vi "StartUp Sequence Open Loop Rev 1.6.vi"() -> ()   [LabVIEW 2017]
uses:
  <vilib>/addons/control/pid/NI_PID_pid.lvlib
  <vilib>/addons/control/pid/pid.llb/PID (DBL).vi
panel:
  in  "Stop":bool
  out "Process variable and Setpoint":cluster{"initial PV":dbl, "SP:":dbl}(graph)
  in  "PID gains":T1={"proportional gain (Kc)"=20.0, "integral time (Ti, min)"=0.008, "derivative time (Td, min)"=0.001} {"derivative time (Td, min)" format="%.3f"; "integral time (Ti, min)" format="%.3f"; "proportional gain (Kc)" format="%.3f"}
  out "Measured RPM:":dbl(slide)=60.754431603254424 scale=0.0..100.0
  in  "Requested RPM:":dbl(slide)=43.790849673202615 min=0.0 max=0.0 scale=0.0..100.0
  out "MV:":dbl(slide)=18.78965245852964 scale=-100.0..100.0
  out "Manipulated variable":i32(graph)
  out "Requested RPM":i32
  out "Waveform Chart":cluster{i32, i32}(graph)
  in  "Set RPM":string
  out "Pump Value 2":string
  in  "Soft Shut Off":bool
  out "Pump Value 1":string
  in  "Send RPM":bool
  in  "Send Command":bool
  in  "Custom Command":string
  out "Startup Success":bool
  in  "Output File":path
  in  "Shut Off":bool
  out "ECU COM Port Out":refnum<visa-resource-name>
  out "Throttle Position":string
  out "Turbine RPM":string
  out "Turbine Temp":string
  out "Error Out":errorcluster
  in  "Error In":errorcluster
  in  "ECU COM Port":refnum<visa-resource-name>
  out "Turbine State":string
  in  "Strt Sqnc":bool
  # "Note: save to a .csv file"
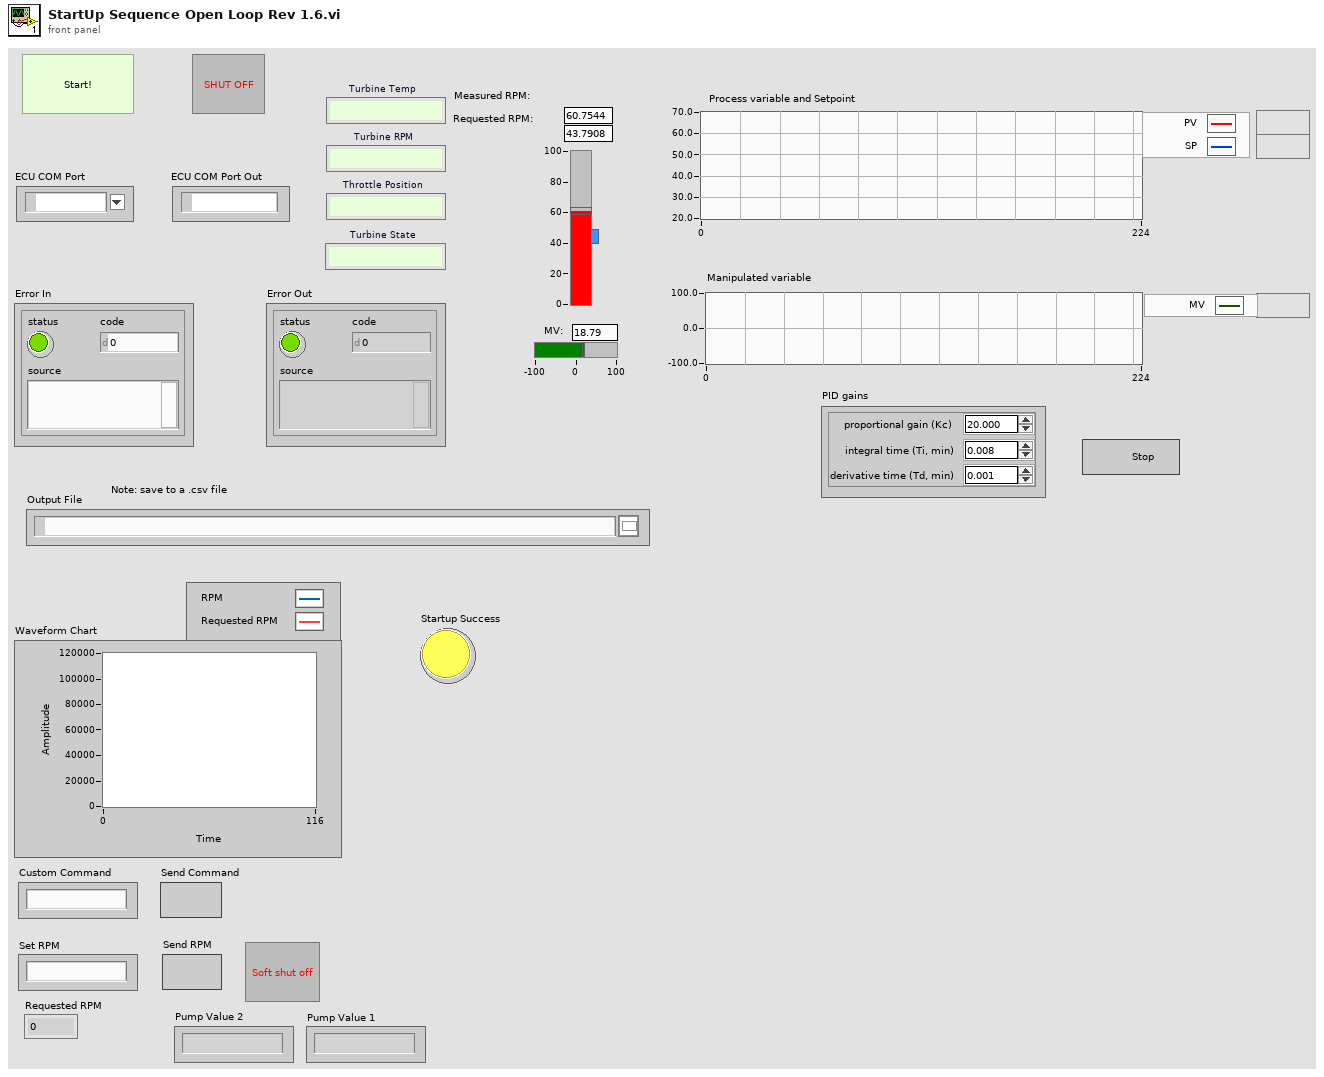
[diagram p1: front panel]
types:
  T1 = cluster{"proportional gain (Kc)":dbl, "integral time (Ti, min)":dbl, "derivative time (Td, min)":dbl}
  T2 = cluster{"Plant Output":dbl, "Requested RPM:":dbl}
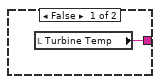
[diagram p4: hidden frame]
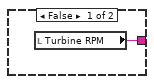
[diagram p5: hidden frame]
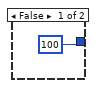
[diagram p7: hidden frame]
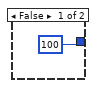
[diagram p8: hidden frame]
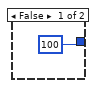
[diagram p9: hidden frame]
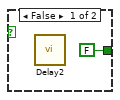
[diagram p11: hidden frame]
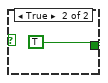
[diagram p12: hidden frame]
diagram:
  w21 = 21 ("Pulse Width")
  w22 = 160 ("Voltage")
  w27 = 16 ("Pulse Width")
  w28 = 160 ("Voltage")
  w18 = 255 ("y")
  w19 = 80 ("y")
  # "NOTE:\nThere are data entry limits\non this input. These may need\nto be deleted in the future"
  # "Disengage Starter Motor"
  # "Starter Motor 55%"
  # "Start button is inside a while loop that doesn't progess until True"
  # "Fuel Pump Mode 2"
  # "GlowPlugOff"
  # "Start Up\nFuelPumpMode 1"
  # "BurnerValveIgnitionPercent"
  # "If False, each Case structure is set\nto an arbitrary Delay time of 0.2 s"
  # "Each Stage is inside a while loop so that \nthe sequence doesn't progress until True"
  n1 = call "Initialize Com Port.vi"("Error In"="Error In", "ECU COM Port"="ECU COM Port") -> ("Error Out"=w38:errorcluster, "ECU COM Port Out"=w37:refnum<visa-resource-name>)  [unwired: 8 in]
  n2 = while {
    tunnel: w38 -> [w135]
    tunnel: [w135] -> w36
    stop <- "Strt Sqnc" stop-if-true
  }
  n3 = call "Initialize Output File.vi"("error in (no error)"=w36, "File Path Control"="Output File") -> ("error out"=w17:errorcluster)  [unwired: 9 in]
  n4 = flat-sequence {
    tunnel: w17 -> [w137]
    tunnel: [w137] -> w32
    frame #0 {
      n5 = local write "Strt Sqnc"(FALSE ("Strt Sqnc")) -> ()
    }
  }
  n6 = flat-sequence {
    tunnel: [w140] -> w16
    tunnel: w17 -> [w140]
    frame #0 {
      w139 = "0" ("Pump Value 1")
      n7 = local write "Pump Value 2"(w139) -> ()
      n8 = local write "Pump Value 1"(w139) -> ()
    }
  }
  n9 = while {
    tunnel: w16 -> [w161]
    tunnel: w37 -> [w160]
    tunnel: "Output File" -> [w157]
    stop <- w156 continue-if-true
    n10 = call "Get Engine Update.vi"("Error In"=w161, "ECU COM Port"=w160) -> ("Error Out"=w158:errorcluster, "Temperature"=w149:string, "RPMs"=w153:string, "ECU COM Port Out"=w155:refnum<visa-resource-name>)  [unwired: 6 in]
    n11 = call "Time Delay4"() -> ()  [unwired: 11 in, 1 out]
    n12 = call "Safety Check.vi"("Temperature"=w149, "RPMs"=w153) -> ("Safe?"=w156:bool)  [unwired: 9 in]
    n13 = Not Equal?(x=w153, y="") -> (x != y?=w151:bool)
    n14 = Not Equal?(x=w149, y="") -> (x != y?=w148:bool)
    n15 = case shown="False" w156 {
      selector: w156 -> [w166 w168]
      tunnel: w155 -> [w167 _]
      tunnel: [w166 w168] -> w154
      frame False {
        n16 = call "Emergency Shutoff.vi"("ECU COM Port"=w167) -> ()  [unwired: 9 in, 2 out]
      }
      frame True {
      }
    }
    n17 = case shown="True" w151 {
      tunnel: w153 -> [_ w165]
      tunnel: [w164 w165] -> w145
      frame False {
        n18 = local read "Turbine RPM"() -> (w164:string)
      }
      frame True {
        "Turbine RPM" <- w165
      }
    }
    n19 = case shown="True" w148 {
      tunnel: w149 -> [_ w163]
      tunnel: [w162 w163] -> w144
      frame False {
        n20 = local read "Turbine Temp"() -> (w162:string)
      }
      frame True {
        "Turbine Temp" <- w163
      }
    }
    n21 = Not(x=w154) -> (.not. x?=w159:bool)
    n22 = Stop(stop? (T)=w159) -> ()
    n23 = local read "Requested RPM"() -> (w142:i32)
    n24 = local read "Pump Value 2"() -> (w146:string)
    n25 = local read "Pump Value 1"() -> (w147:string)
    n26 = Decimal String To Number(string=w145) -> (number=w143:i32)  [unwired: 2 in, 1 out]
    n27 = Bundle(w143, "Requested RPM"=w142) -> (→"Waveform Chart":cluster{i32, "Requested RPM":i32})  [unwired: 1 in]
    n28 = call "Write Data to Output File.vi"("Pump Value 2"=w146, "Pump Value 1"=w147, "Error In"=w158, "Temperature"=w144, "RPM"=w145, "File Path Control"=w157) -> ()  [unwired: 5 in, 1 out]
  }
  n29 = while {
    tunnel: w37 -> [w170]
    tunnel: w38 -> [_]
    stop <- FALSE stop-if-true
    n30 = case shown="True" "Send Command" {
      tunnel: "Custom Command" -> [_ w174]
      tunnel: w170 -> [_ w173]
      frame False {
      }
      frame True {
        n31 = call "Time Delay3"() -> ()  [unwired: 11 in, 1 out]
        n32 = VISA Write(VISA resource name=w173, write buffer=w174) -> ()  [unwired: 1 in, 3 out]
      }
    }
  }
  n33 = flat-sequence {
    tunnel: w32 -> [_]
    frame #0 {
      n34 = local write "Turbine State"("Initializing Motor") -> ()
    }
  }
  n35 = while {
    tunnel: ["Shut Off"] -> w132
    tunnel: "ECU COM Port" -> [w176]
    stop <- "Shut Off" stop-if-true
    # "Turns off each individual component"
    n36 = case shown="True" "Shut Off" {
      tunnel: w176 -> [_ w180]
      frame False {
      }
      frame True {
        n37 = call "Emergency Shutoff.vi"("ECU COM Port"=w180) -> ("Error Out"=w179:errorcluster)  [unwired: 9 in, 1 out]
        n38 = local write "Output File"(path "" ("Output File")) -> ()
        n39 = flat-sequence {
          tunnel: w179 -> [w181]
          tunnel: [w181] -> _
          frame #0 {
            n40 = local write "Strt Sqnc"(FALSE ("Strt Sqnc")) -> ()
          }
        }
      }
    }
  }
  n41 = call "Set Glow Plug Duty Cycle.vi"("Error In"=w32, "Duty Cycle"=6, "ECU COM Port"=w37) -> ("Error Out"=w123:errorcluster, "ECU COM Port Out"=w120:refnum<visa-resource-name>)  [unwired: 7 in]
  n42 = call "Delay"("error in (no error)"=w123) -> ("error out"=w122:errorcluster)  [unwired: 10 in]
  n43 = call "Set Glow Plug Duty Cycle.vi"("Error In"=w122, "Duty Cycle"=19, "ECU COM Port"=w120) -> ("Error Out"=w121:errorcluster, "ECU COM Port Out"=w116:refnum<visa-resource-name>)  [unwired: 7 in]
  n44 = call "Delay"("error in (no error)"=w121) -> ("error out"=w117:errorcluster)  [unwired: 10 in]
  n45 = call "Set Starter Motor Duty Cycle.vi"("Error In"=w117, "Duty Cycle"=6, "ECU COM Port"=w116) -> ("Error Out"=w115:errorcluster, "ECU COM Port Out"=w113:refnum<visa-resource-name>)  [unwired: 7 in]
  n46 = call "Set Glow Plug Duty Cycle.vi"("Error In"=w115, "Duty Cycle"=15, "ECU COM Port"=w113) -> ("Error Out"=w114:errorcluster, "ECU COM Port Out"=w109:refnum<visa-resource-name>)  [unwired: 7 in]
  n47 = call "Delay"("error in (no error)"=w114) -> ("error out"=w111:errorcluster)  [unwired: 10 in]
  n48 = call "Set Starter Motor Duty Cycle.vi"("Error In"=w111, "Duty Cycle"=4, "ECU COM Port"=w109) -> ("Error Out"=w110:errorcluster, "ECU COM Port Out"=w108:refnum<visa-resource-name>)  [unwired: 7 in]
  n49 = call "Delay"("error in (no error)"=w110) -> ("error out"=w133:errorcluster)  [unwired: 10 in]
  n50 = Stop(stop? (T)=w132) -> ()
  n51 = while {
    tunnel: w133 -> [w185]
    tunnel: w108 -> [w184]
    tunnel: [w184] -> w30
    tunnel: [w185] -> w134
    stop <- w188 stop-if-true
    n52 = local read "Turbine RPM"() -> (w183:string)
    n53 = Decimal String To Number(string=w183) -> (number=w187:i32)  [unwired: 2 in, 1 out]
    n54 = Greater Or Equal?(x=w187, y=3300) -> (x >= y?=w189:bool)
    n55 = case shown="True" w189 {
      tunnel: [FALSE TRUE] -> w188
      frame False {
        n56 = call "Delay2"() -> ()  [unwired: 11 in, 1 out]
      }
      frame True {
      }
    }
  }
  n57 = flat-sequence {
    tunnel: w133 -> [_]
    frame #0 {
      n58 = local write "Turbine State"("Stage1 Check RPM") -> ()
    }
  }
  n59 = call "CmdSeparator7"("error in (no error)"=w134) -> ("error out"=w26:errorcluster)  [unwired: 10 in]
  n60 = call "Set Pump Fow Rate.vi"("Error In"=w26, "Pulse Width"=w27, "Voltage"=w28, "ECU COM Port"=w30) -> ("Error Out"=w31:errorcluster, "ECU COM Port Out"=w29:refnum<visa-resource-name>)  [unwired: 6 in]
  n61 = flat-sequence {
    tunnel: w28 -> [w194]
    tunnel: w27 -> [w193]
    tunnel: w26 -> [_]
    frame #0 {
      n62 = Number To Decimal String(number=w193) -> (decimal integer string=w195:string)  [unwired: 1 in]
      n63 = Number To Decimal String(number=w194) -> (decimal integer string=w196:string)  [unwired: 1 in]
      n64 = local write "Pump Value 2"(w195) -> ()
      n65 = local write "Pump Value 1"(w196) -> ()
    }
  }
  n66 = call "CmdSeparator2"("error in (no error)"=w31) -> ("error out"=w107:errorcluster)  [unwired: 10 in]
  n67 = call "Set Burner Valve Percent.vi"("Error In"=w107, "Percent"=10, "ECU COM Port"=w29) -> ("Error Out"=w106:errorcluster, "ECU COM Port Out"=w96:refnum<visa-resource-name>)  [unwired: 7 in]
  n68 = call "CmdSeparator"("error in (no error)"=w106) -> ("error out"=w105:errorcluster)  [unwired: 10 in]
  n69 = call "Set Burner Valve Percent.vi"("Error In"=w105, "Percent"=31, "ECU COM Port"=w96) -> ("Error Out"=w104:errorcluster, "ECU COM Port Out"=w95:refnum<visa-resource-name>)  [unwired: 7 in]
  n70 = call "CmdSeparator10"("error in (no error)"=w104) -> ("error out"=w103:errorcluster)  [unwired: 10 in]
  n71 = call "Set Burner Valve Percent.vi"("Error In"=w103, "Percent"=35, "ECU COM Port"=w95) -> ("Error Out"=w102:errorcluster, "ECU COM Port Out"=w94:refnum<visa-resource-name>)  [unwired: 7 in]
  n72 = call "CmdSeparator11"("error in (no error)"=w102) -> ("error out"=w101:errorcluster)  [unwired: 10 in]
  n73 = call "Set Burner Valve Percent.vi"("Error In"=w101, "Percent"=39, "ECU COM Port"=w94) -> ("Error Out"=w100:errorcluster, "ECU COM Port Out"=w93:refnum<visa-resource-name>)  [unwired: 7 in]
  n74 = call "CmdSeparator12"("error in (no error)"=w100) -> ("error out"=w99:errorcluster)  [unwired: 10 in]
  n75 = call "Set Burner Valve Percent.vi"("Error In"=w99, "Percent"=43, "ECU COM Port"=w93) -> ("Error Out"=w98:errorcluster, "ECU COM Port Out"=w92:refnum<visa-resource-name>)  [unwired: 7 in]
  n76 = call "CmdSeparator13"("error in (no error)"=w98) -> ("error out"=w97:errorcluster)  [unwired: 10 in]
  n77 = call "Set Burner Valve Percent.vi"("Error In"=w97, "Percent"=47, "ECU COM Port"=w92) -> ("Error Out"=w75:errorcluster, "ECU COM Port Out"=w74:refnum<visa-resource-name>)  [unwired: 7 in]
  n78 = call "CmdSeparator6"("error in (no error)"=w75) -> ("error out"=w77:errorcluster)  [unwired: 10 in]
  n79 = call "Set Burner Valve Percent.vi"("Error In"=w77, "Percent"=51, "ECU COM Port"=w74) -> ("Error Out"=w70:errorcluster, "ECU COM Port Out"=w71:refnum<visa-resource-name>)  [unwired: 7 in]
  n80 = call "CmdSeparator8"("error in (no error)"=w70) -> ("error out"=w73:errorcluster)  [unwired: 10 in]
  n81 = call "Set Burner Valve Percent.vi"("Error In"=w73, "Percent"=55, "ECU COM Port"=w71) -> ("Error Out"=w66:errorcluster, "ECU COM Port Out"=w67:refnum<visa-resource-name>)  [unwired: 7 in]
  n82 = call "CmdSeparator14"("error in (no error)"=w66) -> ("error out"=w69:errorcluster)  [unwired: 10 in]
  n83 = call "Set Burner Valve Percent.vi"("Error In"=w69, "Percent"=59, "ECU COM Port"=w67) -> ("Error Out"=w65:errorcluster, "ECU COM Port Out"=w64:refnum<visa-resource-name>)  [unwired: 7 in]
  n84 = call "CmdSeparator9"("error in (no error)"=w65) -> ("error out"=w131:errorcluster)  [unwired: 10 in]
  n85 = flat-sequence {
    tunnel: w131 -> [_]
    frame #0 {
      n86 = local write "Turbine State"("Stage2 Check Temp.") -> ()
    }
  }
  n87 = while {
    tunnel: w64 -> [w199]
    tunnel: w131 -> [w200]
    tunnel: [w199] -> w81
    tunnel: [w200] -> w82
    stop <- w203 stop-if-true
    # "Stage2Temp(C)"
    n88 = local read "Turbine Temp"() -> (w198:string)
    n89 = Decimal String To Number(string=w198) -> (number=w201:i32)  [unwired: 2 in, 1 out]
    n90 = Greater Or Equal?(x=w201, y=90) -> (x >= y?=w204:bool)
    n91 = case shown="False" w204 {
      tunnel: [FALSE TRUE] -> w203
      frame False {
        n92 = call "Delay3"() -> ()  [unwired: 11 in, 1 out]
      }
      frame True {
      }
    }
  }
  n93 = call "Set Glow Plug Duty Cycle.vi"("Error In"=w82, "Duty Cycle"=0, "ECU COM Port"=w81) -> ("Error Out"=w80:errorcluster, "ECU COM Port Out"=w23:refnum<visa-resource-name>)  [unwired: 7 in]
  n94 = call "CmdSeparator3"("error in (no error)"=w80) -> ("error out"=w20:errorcluster)  [unwired: 10 in]
  n95 = call "Set Pump Fow Rate.vi"("Error In"=w20, "Pulse Width"=w21, "Voltage"=w22, "ECU COM Port"=w23) -> ("Error Out"=w25:errorcluster, "ECU COM Port Out"=w24:refnum<visa-resource-name>)  [unwired: 6 in]
  n96 = call "Set Burner Valve Percent.vi"("Error In"=w25, "Percent"=80, "ECU COM Port"=w24) -> ("Error Out"=w63:errorcluster, "ECU COM Port Out"=w78:refnum<visa-resource-name>)  [unwired: 7 in]
  n97 = flat-sequence {
    tunnel: w22 -> [w208]
    tunnel: w21 -> [w207]
    tunnel: w20 -> [_]
    frame #0 {
      n98 = Number To Decimal String(number=w207) -> (decimal integer string=w209:string)  [unwired: 1 in]
      n99 = Number To Decimal String(number=w208) -> (decimal integer string=w210:string)  [unwired: 1 in]
      n100 = local write "Pump Value 2"(w209) -> ()
      n101 = local write "Pump Value 1"(w210) -> ()
    }
  }
  n102 = call "CmdSeparator18"("error in (no error)"=w63) -> ("error out"=w62:errorcluster)  [unwired: 10 in]
  n103 = call "Set Fuel Valve Percent.vi"("Error In"=w62, "Percent"=12, "ECU COM Port"=w78) -> ("Error Out"=w61:errorcluster, "ECU COM Port Out"=w79:refnum<visa-resource-name>)  [unwired: 7 in]
  n104 = call "CmdSeparator16"("error in (no error)"=w61) -> ("error out"=w129:errorcluster)  [unwired: 10 in]
  n105 = for {
    N: 4 -> [_]
    tunnel: [w211] -> _
    tunnel: [w225] -> _
    tunnel: w79 -> [w217]
    tunnel: w129 -> [w218]
    shift-right: [w216] -> w57
    shift-left: 12 -> [w222]
    shift-right: [w213] -> _
    shift-left: 80 -> [w219]
    tunnel: [w225] -> w52 mode=indexing
    tunnel: [w211] -> w58 mode=indexing
    n106 = Less?(x=w222, y=100) -> (x < y?=w223:bool)
    n107 = Less?(x=w219, y=100) -> (x < y?=w220:bool)
    n108 = case shown="True" w220 {
      tunnel: w219 -> [_ w229]
      tunnel: [100 w227] -> w213
      frame False {
      }
      frame True {
        n109 = Add(x=w229, y=5) -> (x+y=w227:i32)
      }
    }
    n110 = case shown="True" w223 {
      tunnel: w222 -> [_ w233]
      tunnel: [100 w231] -> w216
      frame False {
      }
      frame True {
        n111 = Add(x=w233, y=6) -> (x+y=w231:i32)
      }
    }
    n112 = call "Set Fuel Valve Percent.vi"("Error In"=w218, "Percent"=w216, "ECU COM Port"=w217) -> ("Error Out"=w215:errorcluster, "ECU COM Port Out"=w212:refnum<visa-resource-name>)  [unwired: 7 in]
    n113 = call "Set Burner Valve Percent.vi"("Error In"=w215, "Percent"=w213, "ECU COM Port"=w212) -> ("Error Out"=w214:errorcluster, "ECU COM Port Out"=w211:refnum<visa-resource-name>)  [unwired: 7 in]
    n114 = call "CmdSeparator17"("error in (no error)"=w214) -> ("error out"=w225:errorcluster)  [unwired: 10 in]
  }
  n115 = flat-sequence {
    tunnel: w52 -> [_]
    frame #0 {
      n116 = local write "Turbine State"("Pump Ramp Up") -> ()
    }
  }
  n117 = for {
    N: 10 -> [_]
    tunnel: [w241] -> w40
    tunnel: [w252] -> w43
    shift-right: [w248] -> _
    shift-left: w57 -> [w249]
    tunnel: w52 -> [w245] mode=indexing
    tunnel: w58 -> [w244] mode=indexing
    shift-right: [w237] -> w54
    shift-left: 21 -> [w238]
    w236 = 160 ("y")
    n118 = Less?(x=w249, y=100) -> (x < y?=w250:bool)
    n119 = Add(x=w238, y=1) -> (x+y=w237:i32)
    n120 = case shown="True" w250 {
      tunnel: w249 -> [_ w260]
      tunnel: [100 w258] -> w248
      frame False {
      }
      frame True {
        n121 = Add(x=w260, y=5) -> (x+y=w258:i32)
      }
    }
    n122 = call "Set Fuel Valve Percent.vi"("Error In"=w245, "Percent"=w248, "ECU COM Port"=w244) -> ("Error Out"=w247:errorcluster, "ECU COM Port Out"=w246:refnum<visa-resource-name>)  [unwired: 7 in]
    n123 = call "Set Burner Valve Percent.vi"("Error In"=w247, "Percent"=100 ("y"), "ECU COM Port"=w246) -> ("Error Out"=w235:errorcluster, "ECU COM Port Out"=w242:refnum<visa-resource-name>)  [unwired: 7 in]
    n124 = call "Set Pump Fow Rate.vi"("Error In"=w235, "Pulse Width"=w237, "Voltage"=w236, "ECU COM Port"=w242) -> ("Error Out"=w240:errorcluster, "ECU COM Port Out"=w241:refnum<visa-resource-name>)  [unwired: 6 in]
    n125 = flat-sequence {
      tunnel: w236 -> [w254]
      tunnel: w237 -> [w253]
      tunnel: w235 -> [_]
      frame #0 {
        n126 = Number To Decimal String(number=w253) -> (decimal integer string=w255:string)  [unwired: 1 in]
        n127 = Number To Decimal String(number=w254) -> (decimal integer string=w256:string)  [unwired: 1 in]
        n128 = local write "Pump Value 2"(w255) -> ()
        n129 = local write "Pump Value 1"(w256) -> ()
      }
    }
    n130 = call "CmdSeparator20"("error in (no error)"=w240) -> ("error out"=w252:errorcluster)  [unwired: 10 in]
  }
  n131 = call "Set Starter Motor Duty Cycle.vi"("Error In"=w43, "Duty Cycle"=11, "ECU COM Port"=w40) -> ("Error Out"=w42:errorcluster, "ECU COM Port Out"=w41:refnum<visa-resource-name>)  [unwired: 7 in]
  n132 = flat-sequence {
    tunnel: w42 -> [_]
    frame #0 {
      n133 = local write "Turbine State"("Secondary Pump Ramp Up") -> ()
    }
  }
  n134 = for {
    N: 3 -> [_]
    tunnel: [w269] -> w53
    tunnel: [w276] -> w51
    tunnel: w42 -> [w273]
    tunnel: w41 -> [w272]
    shift-right: [w263] -> _
    shift-left: w54 -> [w266]
    w264 = 160 ("y")
    n135 = Add(x=w266, y=10) -> (x+y=w263:i32)
    n136 = call "Set Fuel Valve Percent.vi"("Error In"=w273, "Percent"=100 ("y"), "ECU COM Port"=w272) -> ("Error Out"=w275:errorcluster, "ECU COM Port Out"=w274:refnum<visa-resource-name>)  [unwired: 7 in]
    n137 = call "Set Burner Valve Percent.vi"("Error In"=w275, "Percent"=0 ("y"), "ECU COM Port"=w274) -> ("Error Out"=w262:errorcluster, "ECU COM Port Out"=w270:refnum<visa-resource-name>)  [unwired: 7 in]
    n138 = call "Set Pump Fow Rate.vi"("Error In"=w262, "Pulse Width"=w263, "Voltage"=w264, "ECU COM Port"=w270) -> ("Error Out"=w268:errorcluster, "ECU COM Port Out"=w269:refnum<visa-resource-name>)  [unwired: 6 in]
    n139 = flat-sequence {
      tunnel: w264 -> [w278]
      tunnel: w263 -> [w277]
      tunnel: w262 -> [_]
      frame #0 {
        n140 = Number To Decimal String(number=w277) -> (decimal integer string=w279:string)  [unwired: 1 in]
        n141 = Number To Decimal String(number=w278) -> (decimal integer string=w280:string)  [unwired: 1 in]
        n142 = local write "Pump Value 2"(w279) -> ()
        n143 = local write "Pump Value 1"(w280) -> ()
      }
    }
    n144 = call "CmdSeparator15"("error in (no error)"=w268) -> ("error out"=w276:errorcluster)  [unwired: 10 in]
  }
  n145 = flat-sequence {
    tunnel: w51 -> [_]
    frame #0 {
      n146 = local write "Turbine State"("Hold on to your butts!") -> ()
    }
  }
  n147 = while {
    tunnel: w51 -> [w283]
    tunnel: w53 -> [w282]
    tunnel: [w283] -> w15
    tunnel: [w282] -> w50
    stop <- w284 stop-if-true
    n148 = local read "Turbine RPM"() -> (w287:string)
    n149 = Decimal String To Number(string=w287) -> (number=w286:i32)  [unwired: 2 in, 1 out]
    n150 = Greater?(x=w286, y=30000) -> (0:w284:bool)
  }
  n151 = call "Set Pump Fow Rate.vi"("Error In"=w15, "Pulse Width"=w18, "Voltage"=w19, "ECU COM Port"=w50) -> ("Error Out"=w49:errorcluster, "ECU COM Port Out"=w48:refnum<visa-resource-name>)  [unwired: 6 in]
  n152 = flat-sequence {
    tunnel: w19 -> [w290]
    tunnel: w18 -> [w289]
    tunnel: [w288] -> _
    tunnel: w15 -> [w288]
    frame #0 {
      n153 = Number To Decimal String(number=w289) -> (decimal integer string=w291:string)  [unwired: 1 in]
      n154 = Number To Decimal String(number=w290) -> (decimal integer string=w292:string)  [unwired: 1 in]
      n155 = local write "Pump Value 2"(w291) -> ()
      n156 = local write "Pump Value 1"(w292) -> ()
    }
  }
  n157 = while {
    tunnel: w49 -> [w294]
    tunnel: w48 -> [w293]
    tunnel: [w294] -> w45
    tunnel: [w293] -> w47
    stop <- w295 stop-if-true
    n158 = local read "Turbine RPM"() -> (w298:string)
    n159 = Decimal String To Number(string=w298) -> (number=w297:i32)  [unwired: 2 in, 1 out]
    n160 = Greater?(x=w297, y=44000) -> (0:w295:bool)
  }
  n161 = flat-sequence {
    tunnel: w45 -> [_]
    frame #0 {
      n162 = local write "Turbine State"("Acheived Idle RPM!") -> ()
    }
  }
  n163 = call "Set Starter Motor Duty Cycle.vi"("Error In"=w45, "Duty Cycle"=0, "ECU COM Port"=w47) -> ("Error Out"=w3:errorcluster, "ECU COM Port Out"=w4:refnum<visa-resource-name>)  [unwired: 7 in]
  n164 = flat-sequence {
    tunnel: w3 -> [_]
    frame #0 {
      "Startup Success" <- TRUE
    }
  }
  n165 = while {
    shift-left: 44000.0 ("Plant Output") -> [w312]
    shift-right: _ -> [_]
    tunnel: [w304] -> w2
    tunnel: [w303] -> w1
    tunnel: w4 -> [w301]
    tunnel: w3 -> [w302]
    stop <- "Stop" stop-if-true
    # "If you don't wire dt (s), the PID VI will internally calculate its sampling time. However, this VI will reduce its maximum execution speed since it has some extra calculation. It is always advised to wire dt whenever possible."
    # "Control loop using PID"
    n166 = Wait Until Next ms Multiple(millisecond multiple=u32 50 ("unsigned 32bit integer")) -> ()  [unwired: 1 out]
    n167 = call-poly <vilib>:"PID.vi"("PID gains"="PID gains", "process variable"=w312, "setpoint"="Requested RPM:") -> ("output"=w307:dbl)  [unwired: 7 in, 1 out]
    n168 = Bundle("Plant Output"=w312, "Requested RPM:"="Requested RPM:") -> (→"Process variable and Setpoint":T2)  [unwired: 1 in]
    n169 = call "RPM to Fuel Flow.vi"("Requested RPM"=w307) -> ("Fuel Pump Value 1"=w306:i32)  [unwired: 10 in]
    "MV:" <- w306
    "Manipulated variable" <- w306
    n170 = call "Set Pump Fow Rate.vi"("Error In"=w302, "Pulse Width"=255, "Voltage"=w306, "ECU COM Port"=w301) -> ("Error Out"=w303:errorcluster, "ECU COM Port Out"=w304:refnum<visa-resource-name>)  [unwired: 6 in]
    n171 = local write "Pump Value 2"("255" ("Pump Value 2")) -> ()
    "Measured RPM:" <- w312
  }
  n172 = Decimal String To Number(string="Set RPM") -> (number=w6:i32)  [unwired: 2 in, 1 out]
  n173 = Less?(x=w6, y=135000) -> (x < y?=w12:bool)
  n174 = Greater?(x=w6, y=44000) -> (0:w7:bool)
  n175 = And(x=w7, y=w12) -> (x .and. y?=w10:bool)
  n176 = And(x=w10, y="Send RPM") -> (x .and. y?=w8:bool)
  n177 = case shown="True" w8 {
    tunnel: _ -> [w315 w324]
    tunnel: _ -> [w316 w323]
    tunnel: [w315 w322] -> _
    tunnel: [w316 w321] -> _
    tunnel: w6 -> [_ w317]
    frame False {
    }
    frame True {
      n178 = call "RPM to Fuel Flow.vi"("Requested RPM"=w317) -> ("Fuel Pump Value 1"=w318:i32)  [unwired: 10 in]
      n179 = call "Set Pump Fow Rate.vi"("Error In"=w323, "Pulse Width"=255, "Voltage"=w318, "ECU COM Port"=w324) -> ("Error Out"=w321:errorcluster, "ECU COM Port Out"=w322:refnum<visa-resource-name>)  [unwired: 6 in]
      n180 = Number To Decimal String(number=w318) -> (decimal integer string=→"Pump Value 1":string)  [unwired: 1 in]
      "Requested RPM" <- w317
    }
  }
  n181 = call "Emergency Shutoff.vi"("Error In"=w1, "ECU COM Port"=w2) -> ("Error Out"=w34:errorcluster, "ECU COM Port Out"=→"ECU COM Port Out":refnum<visa-resource-name>)  [unwired: 8 in]
  n182 = call "Time Delay"() -> ()  [unwired: 11 in, 1 out]
  n183 = flat-sequence {
    tunnel: w34 -> [w326]
    tunnel: [w326] -> w130
    frame #0 {
      w325 = "0"
      n184 = local write "Pump Value 1"(w325) -> ()
      n185 = local write "Pump Value 2"(w325) -> ()
    }
  }
  "Error Out" <- w130
